vi "NameYScaleRMS (SubVI).vi"(4 "XYGraph in 2":refnum<vi>, 6 "response unit label 2":string, 7 "response unit label":string, 8 "error in (no error)":errorcluster, 9 "stimulus unit label":string, 10 "XYGraph Refnum in":refnum<vi>, 11 "XYGraph in":refnum<vi>) -> (0 "error out":errorcluster)   [LabVIEW 2018]
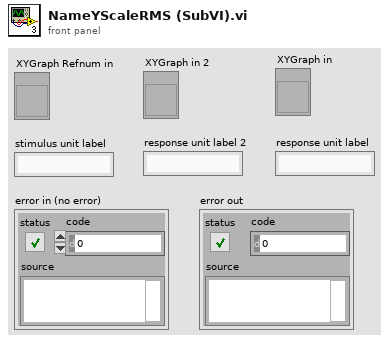
[diagram p1: front panel]
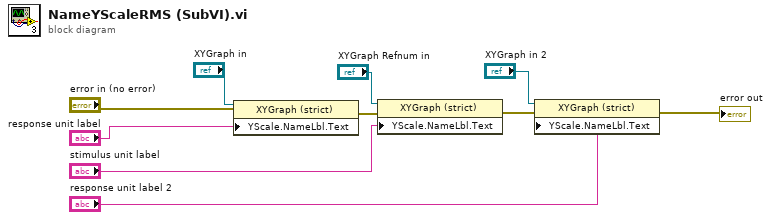
[diagram p0: block diagram]
diagram:
  n1 = property on="Property Node" class="XYGraph (strict)"(reference="XYGraph in", error in="error in (no error)", "YScale.NameLbl.Text"="response unit label") -> (error out=w8:errorcluster)  [unwired: 1 out]
  n2 = property on="Property Node" class="XYGraph (strict)"(reference="XYGraph Refnum in", error in=w8, "YScale.NameLbl.Text"="stimulus unit label") -> (error out=w2:errorcluster)  [unwired: 1 out]
  n3 = property on="Property Node" class="XYGraph (strict)"(reference="XYGraph in 2", error in=w2, "YScale.NameLbl.Text"="response unit label 2") -> (error out=→"error out":errorcluster)  [unwired: 1 out]
